vi "Pre Launch Init.vi"(11 "PublishingModel In":refnum<class "PublishingModel.lvclass">) -> (0 "error out":errorcluster, 3 "PublishingModel Out":refnum<class "PublishingModel.lvclass">)   [LabVIEW 2017, in "TestPubSubRouting.lvlib" / "PublishingModel.lvclass"]
doc: "(<B>Filename</B>: Actor Framework.lvlib:Actor.lvclass:Pre Launch Init.vi)\n\nDefines behavior that occurs after the Launch Nested Actor method is invoked but before the actor's Actor Core method begins running.\n\nBy default, this method does nothing. A descendant class may override it to define behavior."
uses:
  PublishingModel.lvclass
  C:/Git/mva-framework/Source/Framework/IModel/IModel/IModel.lvclass
  <vilib>/ActorFramework/Actor/Actor.lvclass/Actor.ctl
  <vilib>/ActorFramework/Message Enqueuer/Message Enqueuer.lvclass/Message Enqueuer.ctl
  Source/Framework/IModel/IModel/IModel.lvclass/IModel.ctl
  Source/Framework/IMediator/PublishRequest/PublishRequest.lvclass/PublishRequest.ctl
  Source/Framework/AbstractMessages/PreAddressedMsg/PreAddressedMsg.lvclass/PreAddressedMsg.ctl
  Source/Framework/IMediator/IMediator Messages/Publish Msg/Publish Msg.lvclass/Publish Msg.ctl
  Source/Framework/IMediator/IMediator Messages/Publish Msg/Send Pre-Addressed Publish.vi
  Source/Framework/IObserver/IObserver/Read Unique ID.vi
  Source/Framework/IMediator/PublishRequest/Pack Publish Request.vi
  <vilib>/ActorFramework/Message Enqueuer/Enqueue.vi
  Source/Framework/AbstractMessages/PreAddressedMsg/Read Return Address.vi
  <vilib>/ActorFramework/Actor/Read Self Enqueuer.vi
  <vilib>/ActorFramework/Message Enqueuer/Init from Existing Queue.vi
  Source/Framework/IModel/IModel/IModel.lvclass
  C:/Git/mva-framework/Source/Framework/IObserver/IObserver/IObserver.lvclass
  Source/Framework/IObserver/IObserver/IObserver.lvclass
  C:/Program Files (x86)/National Instruments/LabVIEW 2017/vi.lib/ActorFramework/Actor/Actor.lvclass
  Source/Framework/IMediator/IMediator Messages/Publish Msg/Publish Msg.lvclass
  C:/Git/mva-framework/Source/Framework/AbstractMessages/PreAddressedMsg/PreAddressedMsg.lvclass
  C:/Program Files (x86)/National Instruments/LabVIEW 2017/vi.lib/ActorFramework/Message/Message.lvclass
  <vilib>/ActorFramework/Message Priority Queue/Priority Enqueue.vi
  Source/Framework/IMediator/PublishRequest/PublishRequest.lvclass
  <vilib>/ActorFramework/Message Enqueuer/Message Enqueuer.lvclass
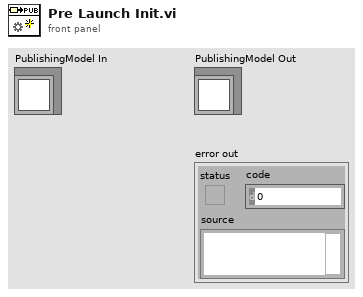
[diagram p1: front panel]
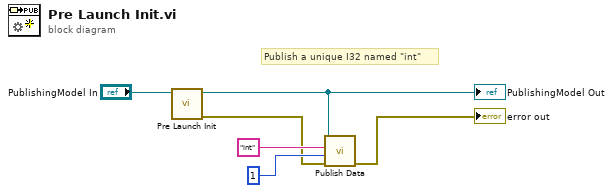
[diagram p0: block diagram]
diagram:
  # "Publish a unique I32 named \"int\""
  n1 = call-parent "Pre Launch Init.vi"("IModel in"="PublishingModel In") -> ("error out"=w2:errorcluster, "IModel out"=w5:refnum<class "PublishingModel.lvclass">)  [unwired: 9 in]
  "PublishingModel Out" <- w5
  n2 = call "Publish Data.vi"("error in (no error)"=w2, "Data to Publish"=1, "Datum Name"="int", "IModel in"=w5) -> ("error out"=→"error out":errorcluster)  [unwired: 6 in, 1 out]
